vi "DAC_V1.vi"() -> ()   [LabVIEW 2020]
uses:
  12e51b78-cc3d-43bc-be07-a567cb738ced.vi
  <vilib>/DAQmx/write.llb/DAQmx Write (Digital 1D Bool NChan 1Samp 1Line).vi
  <vilib>/DAQmx/read.llb/DAQmx Read (Analog 1D Wfm NChan NSamp).vi
  <extravilib>/ChannelInstances/Stream-a[.,.](dbl)/Read With Abort.vi
  <extravilib>/ChannelInstances/Stream-a[.,.](dbl)/Write With Abort.vi
  <extravilib>/ChannelInstances/Stream-a[.,.](dbl)/EndpointRead.vi
  <extravilib>/ChannelInstances/Stream-a[.,.](dbl)/Endpoint.vi
  <vilib>/DAQmx/create/channels.llb/DAQmx Create Channel (AI-Temperature-Thermocouple).vi
  <vilib>/DAQmx/configure/timing.llb/DAQmx Timing (Sample Clock).vi
  <extravilib>/ChannelInstances/Stream-a[.,.](dbl)/Instantiate.vi
  <extravilib>/ChannelInstances/Stream-a[.,.](dbl)/)Channel.vi
  <resource>/ChannelSupport/_ChannelSupport/WaitIfNeeded.vi
  <vilib>/DAQmx/miscellaneous.llb/DAQmx Fill In Error Info.vi
  <resource>/objmgr/daqmx.rc
  <vilib>/ptbypt/NI_PtbyPt.lvlib
  <extravilib>/ChannelInstances/Stream-a[.,.](dbl).lvlib
panel:
  out "Python Reporting Rate (hz)":dbl
  out "Reporting Rate (hz)":dbl
  out "appended array 2":dbl[](array[numeric])
  in  "Purge 2":bool
  in  "Purge 1":bool
  in  "Cycle Fuel":bool
  out "appended array":dbl[][](array[numeric])
  in  "Sensor Stop":bool caption="stop"
  out "TC-CC-430 2":dbl(slide) scale=0.0..500.0
  out "TC-CC-420 2":dbl(slide) scale=0.0..500.0
  out "TC-CC-410 2":dbl(slide) scale=0.0..500.0
  out "TC-OX-260 2":dbl(slide) scale=-350.0..100.0
  out "TC-OC-250 2":dbl(slide) scale=-350.0..100.0
  out "TC-OX-240 2":dbl(slide) scale=-350.0..100.0
  out "TC-OX-230 2":dbl(slide) scale=-350.0..100.0
  out "TC-OX-270 2":dbl(slide) scale=-350.0..100.0
  out "TC-OX-220 2":dbl(slide) scale=-350.0..100.0
  out "TC-OX-210 2":dbl(slide) scale=-350.0..100.0
  out "TC-FU-320 2":dbl(slide) scale=-350.0..100.0
  out "TC-FU-310 2":dbl(slide) scale=0.0..500.0
  in  "Cycle Ox":bool
  in  "Cycle System Sequence":bool
  in  "OXIDIZER GO/NOGO":bool
  in  "FUEL GO/NOGO":bool
  in  "Command GO/NOGO":bool
  in  "Nanny":bool caption="ABORT"
  out "Start Up Time":dbl
  out "IGNITOR STATE":dbl
  out "Nanny":dbl
  in  "Start Up Sequence":bool
  out "Python Input Array":dbl[][](array[numeric])
  out "FM-02":dbl
  out "FM-01":dbl
  in  "file path":path
  in  "Button":bool
  out "current time":timestamp
  in  "FIRE":bool caption="ABORT"
  out "ABORT STATE":dbl
  out "Python Error Out":errorcluster
  in  "ABV-FU-320 (FUEL ISOLATION)":bool
  in  "ABV-OX-240 (LOx MAIN)":bool
  in  "ABV-FU-330 (FUEL PURGE)":bool
  in  "ABV-OX-230 (LOx CHILL)":bool
  in  "ABV-FU-310 (FUEL VENT)":bool
  in  "ABV-OX-220 (LOx ISOLATION)":bool
  in  "ABV-FU-340 (FUEL MAIN)":bool
  in  "ABV-PR-120 (FUEL PRESS)":bool
  in  "ABV-OX-210 (LOx VENT)":bool
  in  "ABV-PR-110 (LOx PRESS)":bool
  in  "ABV-OX-250 (LOx FILL)":bool
  out "Python Returned Valve States":dbl[](array[numeric])
  in  "Python Stop":bool
  in  "ABORT":bool
  out "LabVIEW Error Out":errorcluster
  in  "Error In":errorcluster caption="error in"
  out "PT-SP-520":dbl
  out "PT-SP-510":dbl
  out "Run Tank Voltage FU":dbl
  out "PT-CC-410":dbl
  out "PT-FU-320":dbl
  out "PT-FU-310":dbl
  out "PT-FU-120":dbl
  out "Run Tank Voltage OX":dbl
  out "PT-PR-110":dbl
  out "PT-OX-210":dbl
  out "PT-OX-220":dbl
  out "PT-OX-130":dbl
  out "FUEL Runtank":dbl(slide) scale=0.0..100.0
  out "PT-OX-210 (LOx TANK)":dbl(knob) scale=0.0..1500.0
  out "PT-PR-110 (K-BOTTLE)":dbl(slide) scale=0.0..3500.0
  out "PT-CC-410":dbl(knob) scale=0.0..1500.0
  out "PT-FU-120 (FUEL REGULATOR)":dbl(knob) scale=0.0..3000.0
  out "PT-OX-130 (LOx REGULATOR)":dbl(knob) scale=0.0..3000.0
  out "PT-FU-320 (FUEL MAIN LINE)":dbl(knob) scale=3.0..1500.0
  out "PT-OX-220 (LOx MAIN LINE)":dbl(knob) scale=0.0..1500.0
  out "PT-FU-310 (FUEL TANK)":dbl(knob) scale=0.0..1500.0
  out "Ox Runtank":dbl(slide) scale=0.0..100.0
  # "Spare 1"
  # "Spare 2"
  # "Flow Meter"
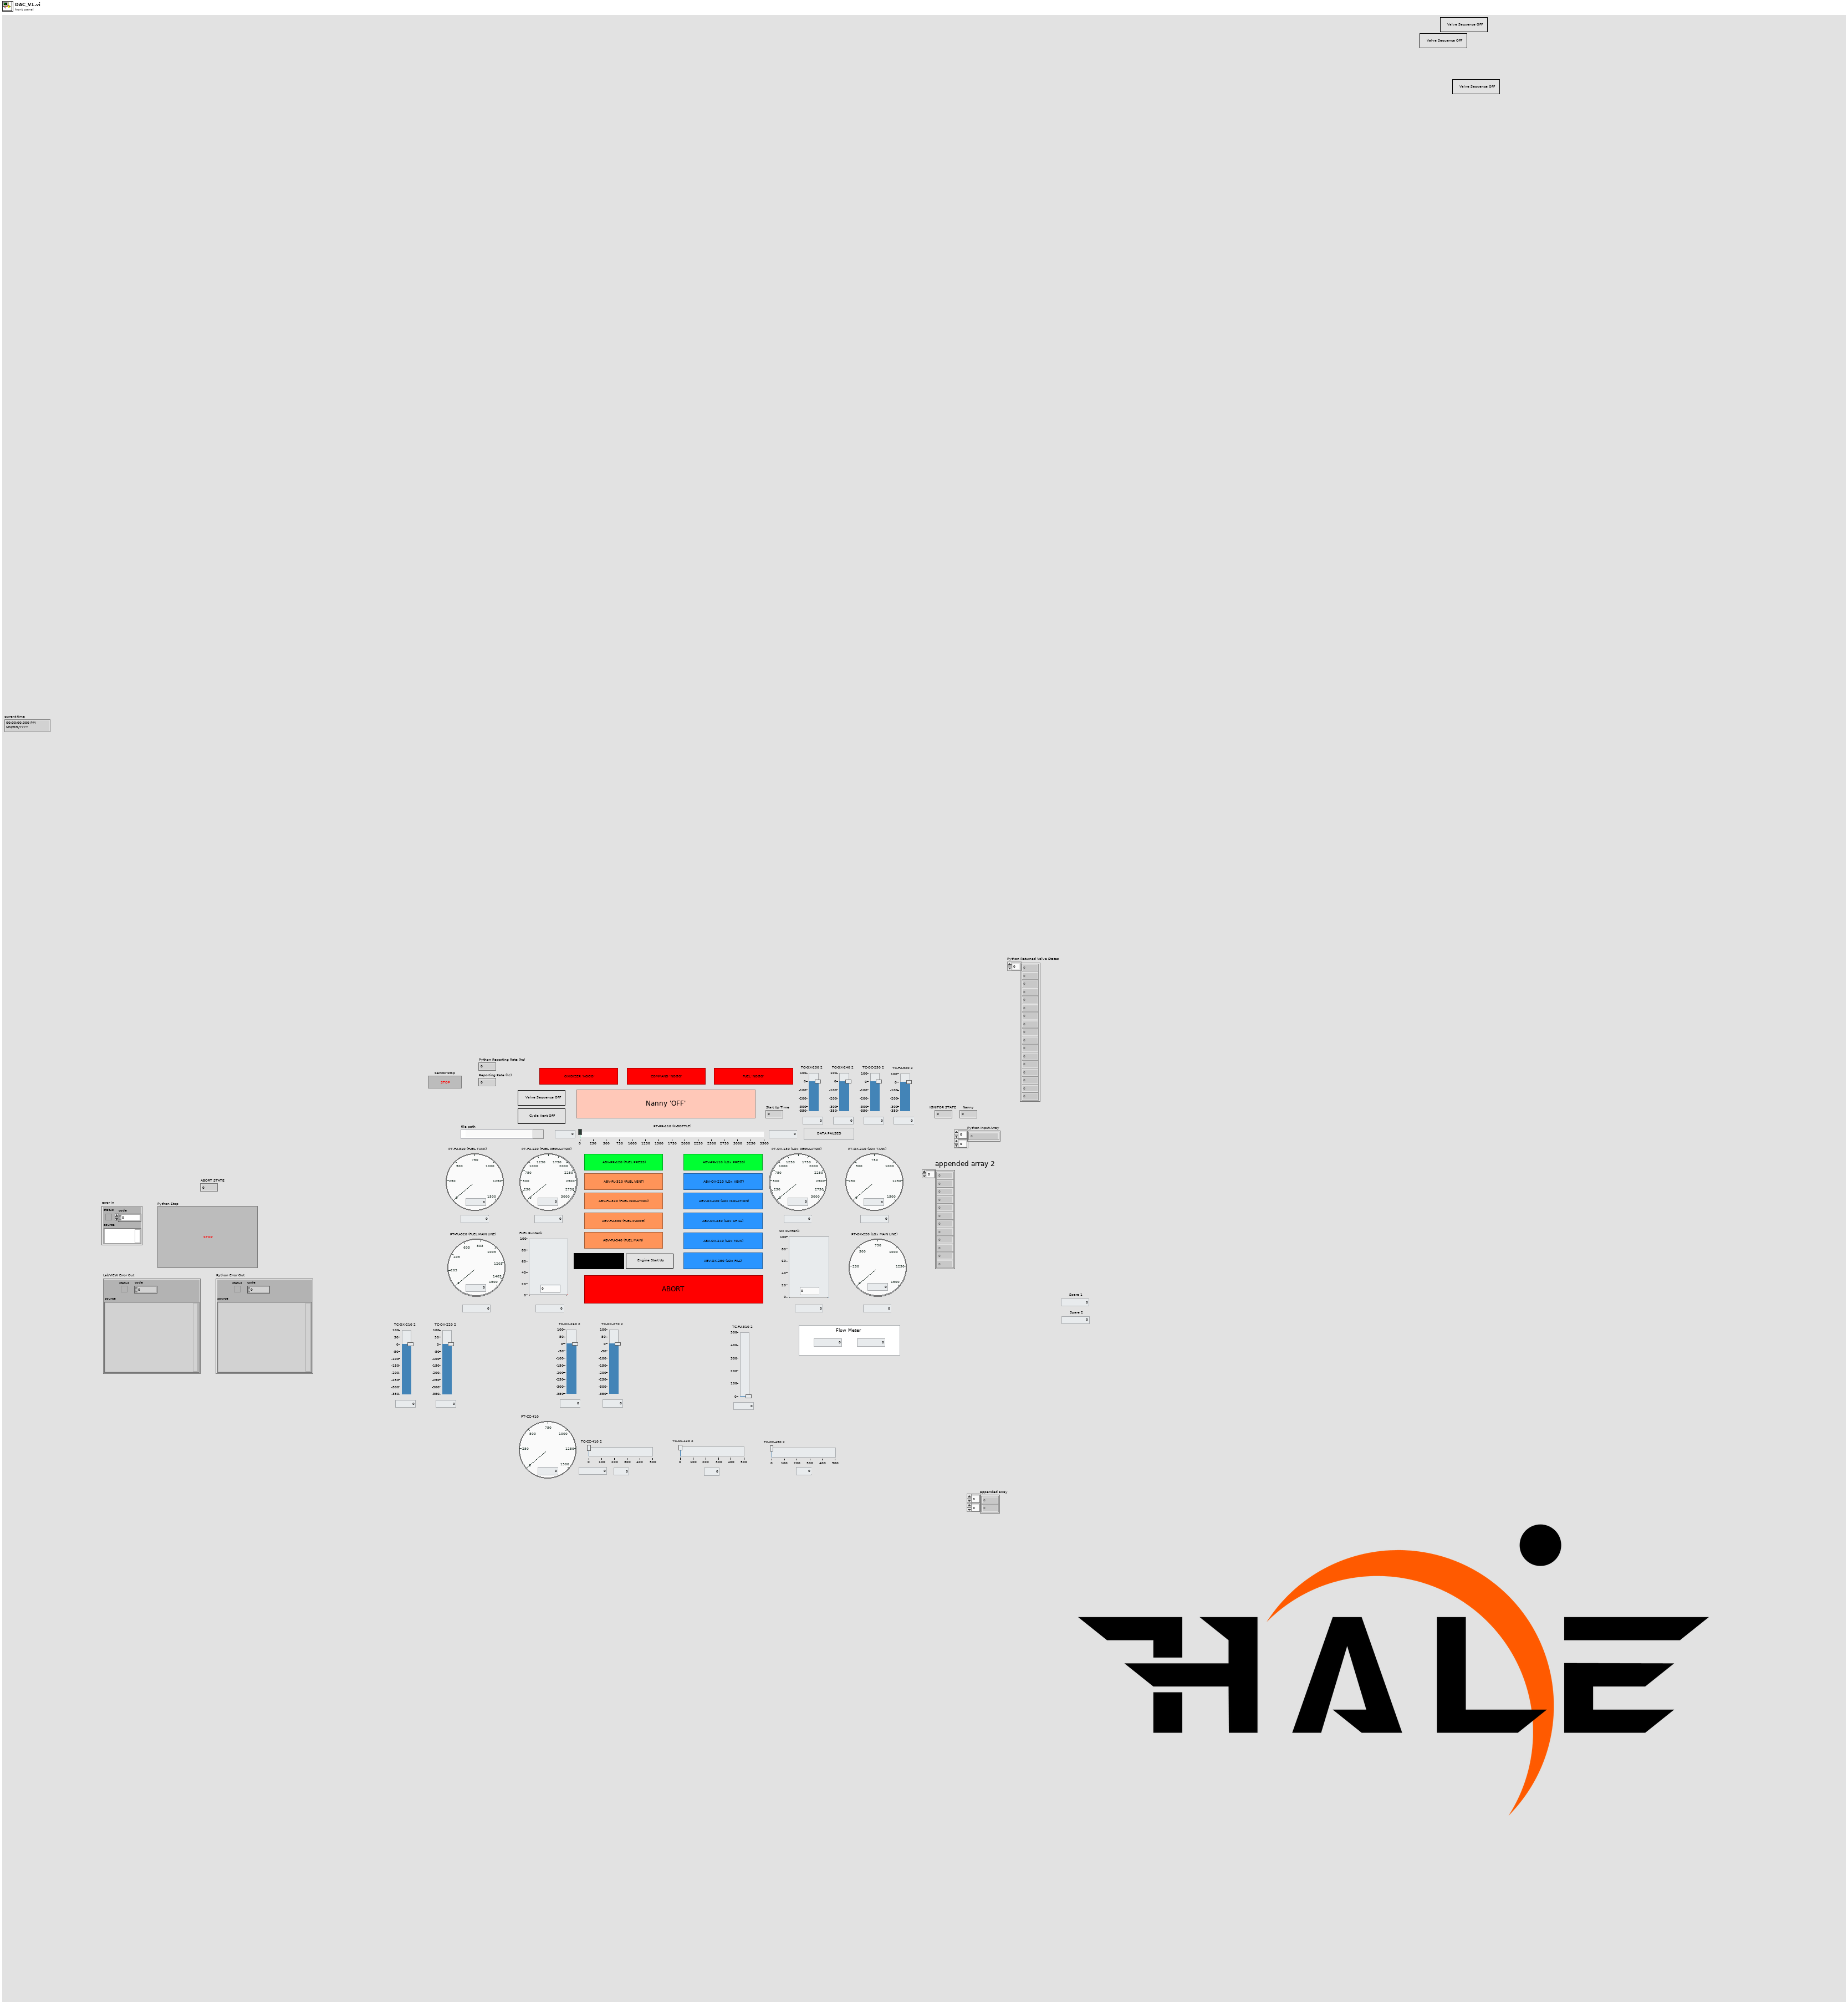
[diagram p1: front panel]
types:
  T1 = enum16{"open", "open or create", "create or replace", "create", "open (read-only)"}
  T2 = typedef "Stream-a[.,.](dbl).lvlib/)Channel.ctl" = refnum<queue>
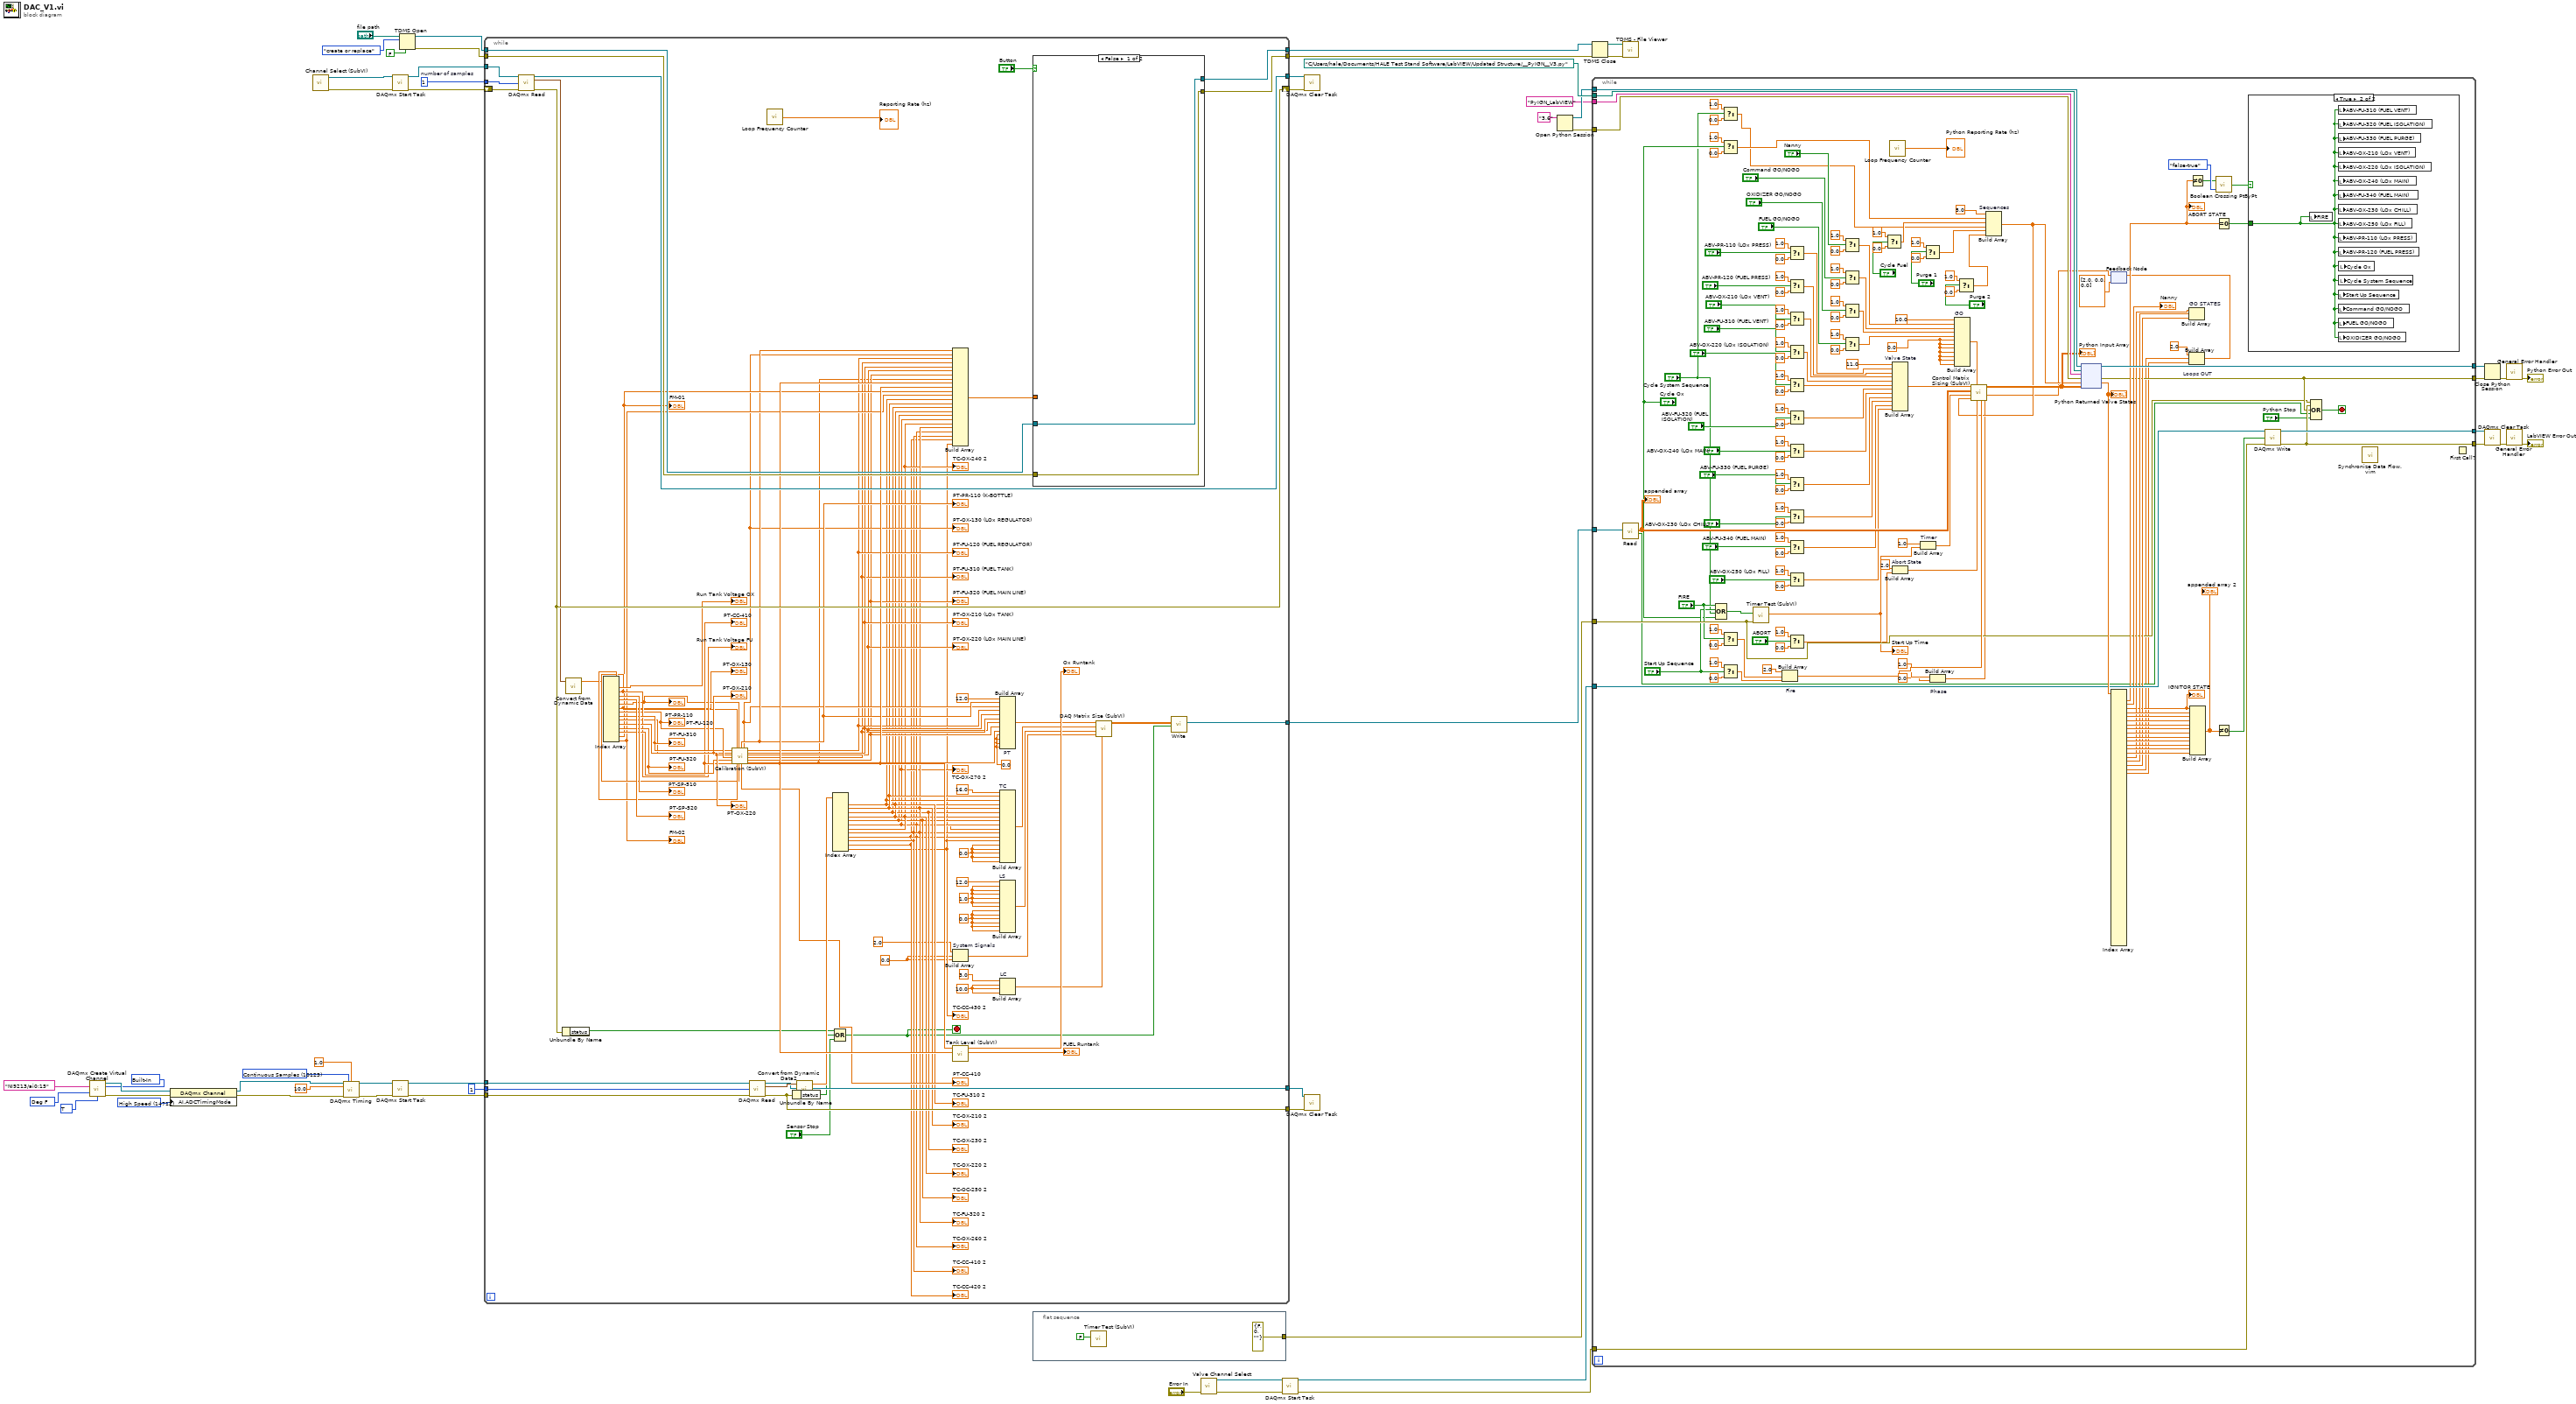
[diagram p0: block diagram]
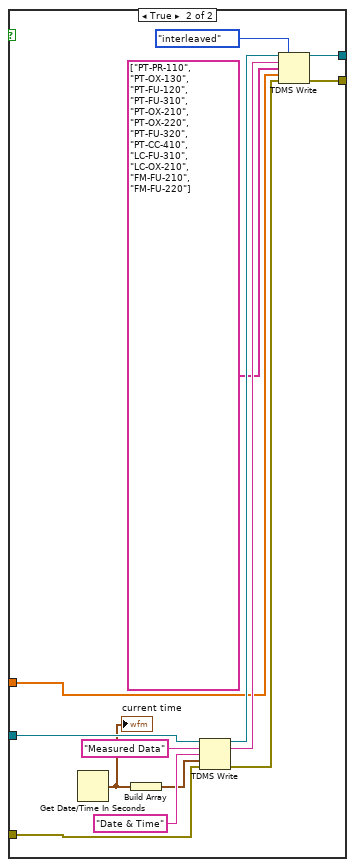
[diagram p3: hidden frame]
diagram:
  w13 = 14712 items=["Automatic"=16097, "High Resolution"=10195, "High Speed"=14712, "Best 50 Hz Rejection"=14713, "Best 60 Hz Rejection"=14714, "Custom"=10137] ("AI.ADCTimingMode")
  w8 = 10200 items=["Built-In"=10200, "Constant Value"=10116, "Channel"=10113] ("cjc source")
  w12 = 10123 items=["Finite Samples"=10178, "Continuous Samples"=10123, "Hardware Timed Single Point"=12522] ("sample mode")
  w6 = 10086 items=["J"=10072, "K"=10073, "N"=10077, "R"=10082, "S"=10085, "T"=10086, "B"=10047, "E"=10055] ("thermocouple type")
  w7 = 10144 items=["Deg C"=10143, "Deg F"=10144, "Kelvins"=10325, "Deg R"=10145, "From Custom Scale"=10065] ("units")
  w53 = 1  # number of samples
  n1 = call-poly <vilib>:"DAQmx Create Virtual Channel.vi"("physical channels"=tag "NI9213/ai0:15", "cjc source"=w8, "units"=w7, "thermocouple type"=w6) -> ("task out"=w16:refnum<k21>, "error out"=w18:errorcluster)  [unwired: 10 in]
  n2 = property class="DAQmx Channel"(reference=w16, error in=w18, "AI.ADCTimingMode"=w13) -> (reference out=w17:refnum<k21>, error out=w19:errorcluster)
  n3 = call "Channel Select (SubVI).vi"() -> ("error out"=w50:errorcluster, "task out"=w49:refnum<k21>)  [unwired: 10 in]
  n4 = call-poly <vilib>:"DAQmx Timing.vi"("task/channels in"=w17, "sample mode"=w12, "samples per channel"=1.0, "rate"=10.0, "error in"=w19) -> ("task out"=w14:refnum<k21>, "error out"=w15:errorcluster)  [unwired: 9 in]
  n5 = call <vilib>:"DAQmx Start Task.vi"("task/channels in"=w49, "error in"=w50) -> ("task out"=w55:refnum<k21>, "error out"=w54:errorcluster)  [unwired: 12 in]
  n6 = call <vilib>:"DAQmx Start Task.vi"("task/channels in"=w14, "error in"=w15) -> ("task out"=w4:refnum<k21>, "error out"=w3:errorcluster)  [unwired: 12 in]
  n7 = TDMS Open(6:FALSE ("disable buffering? (T)"), 10:T1."create or replace" ("operation (0:open)"), 11:"file path") -> (0:w22:errorcluster, 3:w23:refnum<k34>)  [unwired: 4 in]
  n8 = while {
    tunnel: w55 -> [w136]
    tunnel: w53 -> [w133]
    tunnel: [w134] -> w51
    shift-right: [w132] -> w52
    shift-left: w54 -> [w135]
    tunnel: [w120] -> w28
    tunnel: [w119] -> w27
    tunnel: w23 -> [w118]
    tunnel: w22 -> [w117]
    tunnel: [w109] -> w21
    tunnel: 1 ("number of samples per channel") -> [w104]
    tunnel: w4 -> [w103]
    tunnel: w3 -> [w102]
    tunnel: [w101] -> w2
    tunnel: [w100] -> w1
    stop <- w57 stop-if-true
    w59 = 1.0 ("element")
    w61 = 0.0 ("element")
    w63 = 0.0 ("element")
    w64 = 10.0 ("element")
    w82 = 0.0 ("element")
    w78 = 0.0 ("element")
    n9 = call-poly <vilib>:"DAQmx Read.vi"("task/channels in"=w136, "number of samples per channel"=w133, "error in"=w135) -> ("task out"=w134:refnum<k21>, "data"=w66:waveform(dbl)[], "error out"=w132:errorcluster)  [unwired: 10 in]
    n10 = Unbundle By Name(w132) -> ("status"=w99:bool)
    n11 = call "Convert from Dynamic Data"("Dynamic Data Type"=w66) -> ("Array"=w65:dbl[])  [unwired: 3 in]
    n12 = Index Array(array=w65) -> (element #1=w123:dbl, element #2=w122:dbl, element #3=→"PT-SP-510":dbl, element #4=→"PT-SP-520":dbl, element #5=w116:dbl, element #6=w115:dbl, element #7=w114:dbl, element #8=w127:dbl, element #9=w121:dbl, element #10=w126:dbl, element #11=w125:dbl, element #12=w124:dbl, element #13=w111:dbl, element #14=w110:dbl)  [unwired: 14 in]
    "PT-OX-130" <- w115
    "PT-OX-220" <- w126
    "PT-OX-210" <- w121
    "PT-FU-120" <- w114
    "PT-FU-310" <- w127
    "PT-FU-320" <- w125
    "PT-PR-110" <- w116
    "PT-CC-410" <- w124
    "Run Tank Voltage OX" <- w123
    "Run Tank Voltage FU" <- w122
    "FM-01" <- w111
    "FM-02" <- w110
    n13 = call "Calibration (SubVI).vi"("PT-FU-120 (INPUT)"=w114, "PT-OX-210 (INPUT)"=w121, "PT-OX-220 (INPUT)"=w126, "PT-FU-310 (INPUT)"=w127, "PT-FU-320 (INPUT)"=w125, "PT-CC-410 (INPUT)"=w124, "PT-OX-130 (INPUT)"=w115, "LC-OX-210 (INPUT)"=w123, "PT-PR-110 (INPUT)"=w116, "LC-FU-310 (INPUT)"=w122) -> ("PT-PR-110 (OUTPUT)"=w95:dbl, "PT-CC-410 (OUTPUT)"=w88:dbl, "PT-OX-130 (OUTPUT)"=w94:dbl, "LC-FU-310 (OUTPUT)"=w113:dbl, "PT-FU-120 (OUTPUT)"=w93:dbl, "PT-OX-210 (OUTPUT)"=w92:dbl, "PT-OX-220 (OUTPUT)"=w90:dbl, "PT-FU-310 (OUTPUT"=w91:dbl, "PT-FU-320 (OUTPUT)"=w89:dbl, "LC-OX-210 (OUTPUT)"=w112:dbl)
    "PT-FU-310 (FUEL TANK)" <- w91
    "PT-OX-220 (LOx MAIN LINE)" <- w90
    "PT-FU-320 (FUEL MAIN LINE)" <- w89
    "PT-OX-130 (LOx REGULATOR)" <- w94
    "PT-FU-120 (FUEL REGULATOR)" <- w93
    "PT-CC-410" <- w88
    "PT-PR-110 (K-BOTTLE)" <- w95
    "PT-OX-210 (LOx TANK)" <- w92
    n14 = call-poly <vilib>:"DAQmx Read.vi"("task/channels in"=w103, "number of samples per channel"=w104, "error in"=w102) -> ("task out"=w101:refnum<k21>, "data"=w106:waveform(dbl)[], "error out"=w100:errorcluster)  [unwired: 10 in]
    n15 = call "Loop Frequency Counter.vi"() -> ("Loop Rate (Hz)"=→"Reporting Rate (hz)":dbl)
    n16 = Unbundle By Name(w100) -> ("status"=w98:bool)
    n17 = call "Convert from Dynamic Data2"("Dynamic Data Type"=w106) -> ("Array"=w105:dbl[])  [unwired: 3 in]
    n18 = Index Array(array=w105) -> (element #1=w77:dbl, element #2=w79:dbl, element #3=w74:dbl, element #4=w76:dbl, element #5=w72:dbl, element #6=w70:dbl, element #7=w73:dbl, element #8=w75:dbl, element #9=w71:dbl, element #10=w69:dbl, element #11=w68:dbl, element #12=w67:dbl)  [unwired: 12 in]
    "TC-FU-310 2" <- w77
    "TC-FU-320 2" <- w75
    "TC-OX-210 2" <- w79
    "TC-OX-220 2" <- w76
    "TC-OX-270 2" <- w70
    "TC-OX-230 2" <- w74
    "TC-OX-240 2" <- w73
    "TC-OC-250 2" <- w72
    "TC-OX-260 2" <- w71
    "TC-CC-410 2" <- w69
    "TC-CC-420 2" <- w68
    "TC-CC-430 2" <- w67
    n19 = Compound Arithmetic op=OR(w99, w98, "Sensor Stop") -> (w57:bool)
    n20 = Build Array(w95, w94, w93, w91, w92, w90, w89, w88, w113, w112, w111, w110, w77, w79, w74, w76, w72, w70, w73, w75, w71, w69, w68, w67) -> (w107:dbl[])
    n21 = Build Array "System Signals"(2.0 ("element"), w61, w61) -> (w60:dbl[])
    n22 = call "Tank Level (SubVI).vi"("Fuel Tank Input"=w113, "Ox Tank  Input"=w112) -> ("Fuel Tank Output"=→"FUEL Runtank":dbl, "Ox Tank Output"=→"Ox Runtank":dbl)  [unwired: 8 in]
    n23 = Build Array "PT"(12.0 ("element"), w95, w94, w93, w92, w91, w90, w89, w88, w63, w63, w63, w63) -> (w87:dbl[])
    n24 = Build Array "TC"(16.0 ("element"), w79, w77, w76, w75, w74, w73, w72, w71, w70, w69, w68, w67, w78, w78, w78, w78, w78) -> (w84:dbl[])
    n25 = Build Array "LS"(12.0 ("element"), w59, w59, w59, w59, w59, w59, w82, w82, w82, w82, w82, w82) -> (w81:dbl[])
    n26 = Build Array "LC"(3.0 ("element"), w64, w64, w64) -> (w58:dbl[])
    n27 = case shown="False" "Button" {
      tunnel: w118 -> [w138 w149]
      tunnel: w117 -> [w137 w146]
      tunnel: w107 -> [_ w143]
      tunnel: [w138 w142] -> w119
      tunnel: [w137 w141] -> w120
      frame False {
      }
      frame True {
        n28 = Get Date/Time In Seconds() -> (seconds since 1Jan1904=w139:timestamp)
        "current time" <- w139
        n29 = Build Array(w139) -> (w140:timestamp[])
        n30 = TDMS Write(0:w149, 5:"Measured Data" ("group name in (Untitled)"), 7:"Date & Time", 9:w140, 11:w146) -> (4:w152:refnum<k34>, 6:w150:string, 15:w151:errorcluster)  [unwired: 1 in, 1 out]
        n31 = TDMS Write(0:w152, 1:enum16{"decimated", "interleaved"}."interleaved" ("data layout (0:decimated)"), 5:w150, 7:string[] ["PT-PR-110", "PT-OX-130", "PT-FU-120", "PT-FU-310", "PT-OX-210", "PT-OX-220", "PT-FU-320", "PT-CC-410", "LC-FU-310", "LC-OX-210", "FM-FU-210", "FM-FU-220"], 9:w143, 11:w151) -> (4:w142:refnum<k34>, 15:w141:errorcluster)  [unwired: 2 out]
      }
    }
    n32 = call "DAQ Matrix Size (SubVI).vi"("LC Array"=w58, "System Signals"=w60, "LS Array"=w81, "TC Array"=w84, "PT Array"=w87) -> ("Output Matrix"=w86:dbl[][])  [unwired: 6 in]
    n33 = call <extravilib>:"Write.vi"("last element? (F)"=w57, "element"=w86) -> ("channel"=w109:T2)  [unwired: 7 in, 2 out]
  }
  n34 = flat-sequence {
    tunnel: [errorcluster {"status"=FALSE, "code"=0, "source"=""} ("error constant")] -> w20
    frame #0 {
      n35 = call "Timer Test (SubVI).vi"("Boolean"=FALSE) -> ()  [unwired: 9 in, 2 out]
    }
  }
  n36 = call "Valve Channel Select.vi"("error in (no error)"="Error In") -> ("error out"=w44:errorcluster, "Refnum out"=w45:refnum<k21>)  [unwired: 9 in]
  n37 = call <vilib>:"DAQmx Start Task.vi"("task/channels in"=w45, "error in"=w44) -> ("task out"=w43:refnum<k21>, "error out"=w40:errorcluster)  [unwired: 12 in]
  n38 = call <vilib>:"DAQmx Clear Task.vi"("task in"=w51, "error in"=w52) -> ()  [unwired: 13 in, 1 out]
  n39 = call <vilib>:"DAQmx Clear Task.vi"("task in"=w2, "error in"=w1) -> ()  [unwired: 13 in, 1 out]
  n40 = Open Python Session(python version="3.6" ("Python version")) -> (session out=w33:refnum<k35>, error out=w32:errorcluster)  [unwired: 2 in]
  n41 = TDMS Close(8:w28, 11:w27) -> (0:w29:errorcluster, 3:w30:path)
  n42 = while {
    tunnel: w43 -> [w295]
    tunnel: [w312] -> w42
    tunnel: [w273] -> w41
    tunnel: w40 -> [w311]
    tunnel: w32 -> [w307]
    tunnel: w33 -> [w308]
    tunnel: path "C:/Users/hale/Documents/HALE Test Stand Software/LabVIEW/Updated Structure/__PyIGN__V3.py" ("module path") -> [w309]
    tunnel: [w272] -> w37
    tunnel: [w310] -> w36
    tunnel: "PyIGN_LabVIEW" ("function name") -> [w306]
    tunnel: w21 -> [w270]
    tunnel: w20 -> [w262]
    stop <- w274 stop-if-true
    w156 = 0.0 ("element")
    n43 = call <extravilib>:"Read.vi"("channel"=w270) -> ("last element?"=w180:bool, "element"=w263:dbl[][])  [unwired: 6 in, 3 out]
    "appended array" <- w263
    n44 = Compound Arithmetic op=OR("FIRE", "Start Up Sequence", "Cycle System Sequence", "Cycle Ox") -> (w261:bool)
    n45 = Select(t=1.0, s="Cycle System Sequence", f=0.0 ("t")) -> (s? t:f=w165:dbl)
    n46 = Select(t=1.0, s="Cycle Ox", f=0.0 ("t")) -> (s? t:f=w170:dbl)
    n47 = Select(t=1.0, s="FIRE", f=0.0 ("t")) -> (s? t:f=w202:dbl)
    n48 = Select(t=1.0, s="Start Up Sequence", f=0.0 ("t")) -> (s? t:f=w201:dbl)
    n49 = call "Timer Test (SubVI).vi"("Error In"=w262, "Boolean"=w261) -> ("t"=w260:dbl)  [unwired: 8 in, 1 out]
    "Start Up Time" <- w260
    n50 = Build Array "Fire"(2.0 ("element"), w202, w201) -> (w265:dbl[])
    n51 = Select(t=1.0, s="ABV-PR-110 (LOx PRESS)", f=0.0 ("t")) -> (s? t:f=w253:dbl)
    n52 = Select(t=1.0, s="ABV-PR-120 (FUEL PRESS)", f=0.0 ("t")) -> (s? t:f=w194:dbl)
    n53 = Select(t=1.0, s="ABV-OX-210 (LOx VENT)", f=0.0 ("t")) -> (s? t:f=w193:dbl)
    n54 = Select(t=1.0, s="ABV-FU-310 (FUEL VENT)", f=0.0 ("t")) -> (s? t:f=w256:dbl)
    n55 = Select(t=1.0, s="ABV-OX-220 (LOx ISOLATION)", f=0.0 ("t")) -> (s? t:f=w211:dbl)
    n56 = Select(t=1.0, s="ABV-FU-320 (FUEL ISOLATION)", f=0.0 ("t")) -> (s? t:f=w209:dbl)
    n57 = Select(t=1.0, s="ABV-OX-240 (LOx MAIN)", f=0.0 ("t")) -> (s? t:f=w207:dbl)
    n58 = Select(t=1.0, s="ABV-FU-330 (FUEL PURGE)", f=0.0 ("t")) -> (s? t:f=w205:dbl)
    n59 = Select(t=1.0, s="ABV-OX-230 (LOx CHILL)", f=0.0 ("t")) -> (s? t:f=w213:dbl)
    n60 = Select(t=1.0, s="ABV-FU-340 (FUEL MAIN)", f=0.0 ("t")) -> (s? t:f=w214:dbl)
    n61 = Select(t=1.0, s="ABV-OX-250 (LOx FILL)", f=0.0 ("t")) -> (s? t:f=w216:dbl)
    n62 = Select(t=1.0, s="ABORT", f=0.0 ("t")) -> (s? t:f=w197:dbl)
    n63 = Select(t=1.0, s="Nanny", f=0.0 ("t")) -> (s? t:f=w184:dbl)
    n64 = Select(t=1.0, s="Command GO/NOGO", f=0.0 ("t")) -> (s? t:f=w186:dbl)
    n65 = Select(t=1.0, s="OXIDIZER GO/NOGO", f=0.0 ("t")) -> (s? t:f=w189:dbl)
    n66 = Select(t=1.0, s="FUEL GO/NOGO", f=0.0 ("t")) -> (s? t:f=w191:dbl)
    n67 = Select(t=1.0, s="Cycle Fuel", f=0.0 ("t")) -> (s? t:f=w167:dbl)
    n68 = call "Loop Frequency Counter.vi"() -> ("Loop Rate (Hz)"=→"Python Reporting Rate (hz)":dbl)
    n69 = Build Array "Valve State"(11.0 ("element"), w253, w194, w193, w256, w211, w209, w207, w205, w213, w214, w216) -> (w267:dbl[])
    n70 = Build Array "Abort State"(2.0 ("element"), w197) -> (w269:dbl[])
    n71 = Build Array "Timer"(1.0 ("element"), w260) -> (w268:dbl[])
    n72 = Select(t=1.0, s="Purge 1", f=0.0 ("t")) -> (s? t:f=w161:dbl)
    n73 = Build Array "Phase"(1.0 ("element"), 0.0 ("element")) -> (w171:dbl[])
    n74 = Build Array "GO"(10.0 ("element"), w184, w186, w189, w191, w156, w156, w156, w156, w156, w156, w156) -> (w266:dbl[])
    n75 = Select(t=1.0, s="Purge 2", f=0.0 ("t")) -> (s? t:f=w157:dbl)
    n76 = Build Array "Sequences"(5.0 ("element"), w170, w167, w165, w161, w157) -> (w181:dbl[])
    n77 = feedback #1(dbl[] [2.0, 0.0, 0.0]) -> (w174:dbl[])
    n78 = call "Control Matrix Sizing (SubVI).vi"("Phase"=w171, "Loops"=w174, "Fire/Startup"=w265, "Abort State"=w269, "GO States"=w266, "Sequences"=w181, "Timer"=w268, "Input Matrix"=w263, "Valve States"=w267) -> ("Output Matrix"=w264:dbl[][])  [unwired: 2 in]
    "Python Input Array" <- w264
    n79 = node(w308, w309, w306, w307, w181, w264) -> (w310:refnum<k35>, w272:errorcluster, w305:dbl[])  [unwired: 1 in, 2 out]
    "Python Returned Valve States" <- w305
    n80 = Index Array(array=w305) -> (element #1=w283:dbl, element #2=→"Nanny":dbl, element #3=w286:dbl, element #4=w304:dbl, element #5=w303:dbl, element #6=w302:dbl, element #7=w301:dbl, element #8=w300:dbl, element #9=w299:dbl, element #10=w298:dbl, element #11=w297:dbl, element #12=w294:dbl, element #13=w293:dbl, element #14=w292:dbl, element #15=w289:dbl, element #16=w290:dbl, element #17=w288:dbl, element #18=w178:dbl, element #19=w179:dbl)  [unwired: 61 in, 42 out]
    "ABORT STATE" <- w283
    "IGNITOR STATE" <- w286
    n81 = Build Array "GO STATES"(w289, w290, w288) -> ()  [unwired: 1 out]
    n82 = Build Array "Loops OUT"(2.0 ("element"), w178, w179) -> (w176:dbl[])
    n83 = feedback-in #1(w176) -> ()
    n84 = Build Array(w286, w304, w303, w302, w301, w300, w299, w298, w297, w294, w293, w292) -> (w287:dbl[])
    "appended array 2" <- w287
    n85 = Not Equal To 0?(x=w283) -> (x != 0?=w281:bool)
    n86 = call <vilib>:"Boolean Crossing PtByPt.vi"("direction"=enum16{"either", "false-true", "true-false"}."false-true", "input"=w281) -> ("crossing"=w285:bool)  [unwired: 1 in]
    n87 = Equal To 0?(x=w283) -> (x = 0?=w282:bool)
    n88 = Not Equal To 0?(x=w287) -> (x != 0?=w296:bool[])
    n89 = case shown="True" w285 {
      tunnel: w282 -> [_ w313]
      frame False {
      }
      frame True {
        n90 = local write "FIRE"(w313) -> ()
        n91 = local write "ABV-FU-310 (FUEL VENT)"(w313) -> ()
        n92 = local write "ABV-FU-320 (FUEL ISOLATION)"(w313) -> ()
        n93 = local write "ABV-FU-330 (FUEL PURGE)"(w313) -> ()
        n94 = local write "ABV-OX-210 (LOx VENT)"(w313) -> ()
        n95 = local write "ABV-OX-220 (LOx ISOLATION)"(w313) -> ()
        n96 = local write "ABV-OX-240 (LOx MAIN)"(w313) -> ()
        n97 = local write "ABV-FU-340 (FUEL MAIN)"(w313) -> ()
        n98 = local write "ABV-OX-230 (LOx CHILL)"(w313) -> ()
        n99 = local write "ABV-OX-250 (LOx FILL)"(w313) -> ()
        n100 = local write "ABV-PR-110 (LOx PRESS)"(w313) -> ()
        n101 = local write "ABV-PR-120 (FUEL PRESS)"(w313) -> ()
        n102 = local write "Start Up Sequence"(w313) -> ()
        n103 = local write "Command GO/NOGO"(w313) -> ()
        n104 = local write "FUEL GO/NOGO"(w313) -> ()
        n105 = local write "OXIDIZER GO/NOGO"(w313) -> ()
        n106 = local write "Cycle Ox"(w313) -> ()
        n107 = local write "Cycle System Sequence"(w313) -> ()
      }
    }
    n108 = call-poly <vilib>:"DAQmx Write.vi"("task/channels in"=w295, "data"=w296, "error in"=w311) -> ("task out"=w312:refnum<k21>, "error out"=w273:errorcluster)  [unwired: 10 in, 1 out]
    n109 = Compound Arithmetic op=OR(w262, w273, w272, w180, "Python Stop") -> (w274:bool)
    n110 = call "Synchronize Data Flow.vim"() -> ()  [unwired: 4 in, 4 out]
    n111 = First Call?() -> ()  [unwired: 1 out]
  }
  n112 = call <vilib>:"TDMS - File Viewer.vi"("error in (no error)"=w29, "file path"=w30) -> ()  [unwired: 4 in, 2 out]
  n113 = Close Python Session(session in=w36, error in=w37) -> (11:w34:errorcluster)
  n114 = call <vilib>:"DAQmx Clear Task.vi"("task in"=w42, "error in"=w41) -> ("error out"=w47:errorcluster)  [unwired: 13 in]
  n115 = call <vilib>:"General Error Handler.vi"("error in (no error)"=w34) -> ("error out"=→"Python Error Out":errorcluster)  [unwired: 10 in, 4 out]
  n116 = call <vilib>:"General Error Handler.vi"("error in (no error)"=w47) -> ("error out"=→"LabVIEW Error Out":errorcluster)  [unwired: 10 in, 4 out]
